vi "APP1 SHARE.vi"() -> ()   [LabVIEW 2017]
panel:
  in  "stop":bool
  in  "shared variable refnum in":refnum<k21>
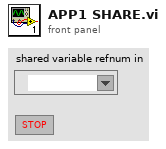
[diagram p1: front panel]
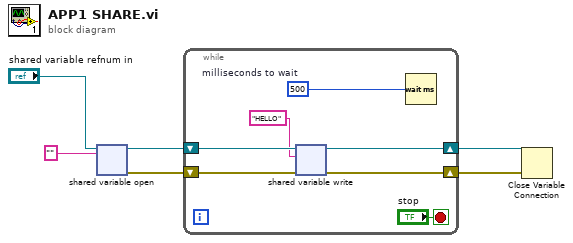
[diagram p0: block diagram]
diagram:
  n1 = shared-variable-open("shared variable refnum in", "") -> (w6:refnum<k21>, w4:errorcluster)  [unwired: 2 in]
  n2 = while {
    shift-right: [w12] -> w5
    shift-left: w6 -> [w13]
    shift-right: [w10] -> w3
    shift-left: w4 -> [w11]
    stop <- "stop" stop-if-true
    w7 = u32 500  # milliseconds to wait
    n3 = shared-variable-write(w13, w11, "HELLO") -> (w12:refnum<k21>, w10:errorcluster)
    n4 = Wait (ms)(milliseconds to wait=w7) -> ()  [unwired: 1 out]
  }
  n5 = Close Variable Connection(8:w3, 11:w5) -> ()  [unwired: 1 out]
